vi "Lab Panel V5.22.vi"() -> ()   [LabVIEW 2013] (continued)
                      tunnel: w836 -> [_ w852]
                      tunnel: w835 -> [_ w851]
                      tunnel: w834 -> [_ w850]
                      tunnel: w833 -> [w843 w849]
                      tunnel: w832 -> [_ w847]
                      frame #0 {
                        n568 = Unbundle(w843) -> ("AMPS"=w846:dbl)  [unwired: 4 out]
                        n569 = call "Check For Amps on v1.vi"("ID"="LAB01-2", "amps"=w846) -> ("amps"=w844:bool)  [unwired: 9 in]
                      }
                      frame #1 {
                        n570 = case shown="True" w848 {
                          tunnel: w858 -> [_ w871]
                          tunnel: w857 -> [_ w870]
                          tunnel: w856 -> [_ w869]
                          tunnel: w855 -> [_ w868]
                          tunnel: w854 -> [_ w867]
                          tunnel: [errorcluster {"status"=FALSE, "code"=0, "source"=""} ("error out") w866] -> w853
                          tunnel: w852 -> [_ w865]
                          tunnel: w851 -> [_ w864]
                          tunnel: w850 -> [_ w863]
                          tunnel: w849 -> [_ w862]
                          tunnel: w847 -> [_ w861]
                          frame False {
                            w859 = FALSE
                            n571 = local write "RUN LAB01-2"(w859) -> ()
                            n572 = local write "run lab01-2"(w859) -> ()
                          }
                          frame True {
                            n573 = stacked-sequence {
                              seq-local: [w872 _ _ _ _] -> [_ w896 _ _ _]
                              tunnel: w871 -> [w877 _ _ _ _]
                              tunnel: w870 -> [w874 _ _ _ _]
                              tunnel: w869 -> [w887 _ _ _ _]
                              tunnel: w868 -> [w880 _ _ _ _]
                              tunnel: w867 -> [w875 _ _ _ _]
                              tunnel: [_ w891 _ _ _] -> w866
                              tunnel: w865 -> [_ _ _ w918 _]
                              tunnel: w864 -> [_ _ _ w917 _]
                              tunnel: w863 -> [_ _ _ w916 _]
                              tunnel: w862 -> [_ _ _ _ _]
                              tunnel: w861 -> [_ _ _ _ w931]
                              frame #0 {
                                w873 = "\\"
                                n574 = local read "SET LAB01-2"() -> (w882:T5)
                                n575 = case shown="\"CYCLE TEST\"" w887 {
                                tunnel: ["L01-2-CHART TEST-" "L01-2-CYCLE TEST-" "L01-2-T-RISE TEST-"] -> w883
                                frame "CHART TEST", Default {
                                }
                                frame "CYCLE TEST" {
                                }
                                frame "T-RISE TEST" {
                                }
                                }
                                n576 = Unbundle(w882) -> ("DESCRIPTION"=w881:string)  [unwired: 4 out]
                                n577 = Concatenate Strings(w877, "\\", w875, w873, w874, w873) -> (w884:string)
                                n578 = String To Path(string=w884) -> (path=w886:path)
                                n579 = Concatenate Strings(w884, w883, w881, "-", w880, ".tdms") -> (w872:string)
                                n580 = Create Folder(path (use dialog)=w886) -> (error out=w885:errorcluster)  [unwired: 2 in, 2 out]
                                n581 = call <vilib>:"Clear Errors.vi"("error in (no error)"=w885) -> ()  [unwired: 6 in, 1 out]
                                n582 = global write "Global 1.vi" "LAB01-2 FILE"(w872) -> ()
                              }
                              frame #1 {
                                (unwired) FALSE
                                n583 = String To Path(string=w896) -> (path=w892:path)
                                n584 = TDMS Open(6:FALSE, 10:T20."create or replace" ("operation (0:open)"), 11:w892) -> (0:w891:errorcluster, 3:→"TDMS LAB01-2":refnum<k34>)  [unwired: 4 in]
                              }
                              frame #2 {
                                n585 = local read "SET LAB01-2"() -> (w902:T5)
                                n586 = local read "TDMS LAB01-2"() -> (w913:refnum<k34>)
                                n587 = Build Array("Testers Name", "Description", "Set Test Cycles", "T-Rise minutes", "T-Rise Deg C") -> (w903:string[])
                                n588 = Unbundle(w902) -> ("NAME"=w901:string, "DESCRIPTION"=w900:string, "CYCLES"=w899:dbl, "T-RISE mins"=w898:dbl, "T-RISE deg C"=w897:dbl)
                                n589 = Number To Decimal String(number=w899) -> (decimal integer string=w912:string)  [unwired: 1 in]
                                n590 = Number To Decimal String(number=w898) -> (decimal integer string=w911:string)  [unwired: 1 in]
                                n591 = Number To Decimal String(number=w897) -> (decimal integer string=w910:string)  [unwired: 1 in]
                                n592 = Build Array(w901, w900, w912, w911, w910) -> (w909:string[])
                                n593 = TDMS Set Properties(5:w909, 7:w903, 11:w913) -> ()  [unwired: 3 in, 4 out]
                              }
                              frame #3 {
                                n594 = local read "DISP LAB01-2"() -> (w915:T4)
                                n595 = Concatenate Strings("LAB01-2  ", w918) -> (w919:string)
                                n596 = Two Button Dialog(message=w919, 1:w916, 2:w917) -> (T button?=w921:bool)
                                n597 = case shown="True" w921 {
                                tunnel: w915 -> [w928 w929]
                                tunnel: [w928 w929] -> w925
                                tunnel: [w927 w930] -> w924
                                tunnel: [w926 w930] -> w923
                                frame False {
                                n598 = Unbundle(w928) -> ("CYCLE"=w927:dbl, "MINS"=w926:dbl)  [unwired: 1 out]
                                }
                                frame True {
                                w930 = 0.0
                                }
                                }
                                n599 = Bundle(cluster=w925, "CYCLE"=w924, "MINS"=w923, "STATUS"="RUN") -> (w914:T4)
                                n600 = local write "DISP LAB01-2"(w914) -> ()
                              }
                              frame #4 {
                                n601 = local read "TEMP START LAB01-2"() -> (w933:cluster{"TL":dbl, "TN":dbl})
                                n602 = Bundle(cluster=w933, "TL"=w931, "TN"=w931) -> (w932:cluster{"TL":dbl, "TN":dbl})
                                n603 = local write "TEMP START LAB01-2"(w932) -> ()
                              }
                            }
                          }
                        }
                      }
                    }
                  }
                }
              }
              event "RUN LAB02-1": Value Change {
                n604 = event-data() -> ("NewVal"=w939:bool)  [unwired: 1 in, 5 out]
                n605 = local read "SIG LAB02-1"() -> (w935:T2)
                n606 = case shown="True" w939 {
                  tunnel: w945 -> [_ w983]
                  tunnel: w944 -> [_ w982]
                  tunnel: w942 -> [w947 w981]
                  tunnel: w943 -> [_ w980]
                  tunnel: w941 -> [_ w979]
                  tunnel: [w946 w978] -> w940
                  tunnel: w938 -> [_ w977]
                  tunnel: w937 -> [_ w976]
                  tunnel: w936 -> [_ w975]
                  tunnel: w935 -> [_ w974]
                  tunnel: w934 -> [_ w973]
                  frame False {
                    # "stop test"
                    n607 = stacked-sequence {
                      tunnel: w947 -> [w956 _]
                      tunnel: [w948 _] -> w946
                      frame #0 {
                        n608 = local read "DISP LAB02-1"() -> (w955:T4)
                        n609 = Unbundle(w955) -> ("CYCLE"=w953:dbl, "MINS"=w954:dbl)  [unwired: 1 out]
                        n610 = case shown="\"CYCLE TEST\"" w956 {
                          tunnel: w954 -> [_ _ w963]
                          tunnel: w953 -> [w961 w962 _]
                          tunnel: [w961 w962 w963] -> w952
                          frame "CHART TEST", Default {
                          }
                          frame "CYCLE TEST" {
                          }
                          frame "T-RISE TEST" {
                          }
                        }
                        n611 = local read "TDMS LAB02-1"() -> (w960:refnum<k34>)
                        n612 = Build Array("STOPPED") -> (w957:string[])
                        n613 = Build Array(w952) -> (w951:dbl[])
                        n614 = TDMS Write(0:w960, 5:"TEST RESULT", 7:w957, 9:w951) -> (4:w949:refnum<k34>, 15:w950:errorcluster)  [unwired: 2 in, 2 out]
                        n615 = TDMS Close(8:w950, 11:w949) -> (0:w948:errorcluster)  [unwired: 1 out]
                      }
                      frame #1 {
                        n616 = local read "DISP LAB02-1"() -> (w967:T4)
                        n617 = stacked-sequence {
                          tunnel: "LAB02-1" -> [w969 w971]
                          frame #0 {
                            n618 = call "sub vi - defrag tdms v1.vi"("panel id"=w969) -> ("error out"=w968:errorcluster)  [unwired: 10 in]
                            n619 = local write "data file error"(w968) -> ()
                          }
                          frame #1 {
                            n620 = local write "RESULT LAB02-1"(FALSE) -> ()
                            n621 = call "Save data file (stop) v3.vi"("panel id"=w971) -> ("network file save error"=w970:errorcluster)  [unwired: 9 in, 1 out]
                            n622 = local write "data file error"(w970) -> ()
                          }
                        }
                        n623 = Bundle(cluster=w967, "STATUS"="STOP") -> (w965:T4)  [unwired: 2 in]
                        n624 = local write "DISP LAB02-1"(w965) -> ()
                      }
                    }
                  }
                  frame True {
                    n625 = stacked-sequence {
                      seq-local: [w985 _] -> [_ w989]
                      tunnel: w983 -> [_ w999]
                      tunnel: w982 -> [_ w998]
                      tunnel: w981 -> [_ w997]
                      tunnel: w980 -> [_ w996]
                      tunnel: w979 -> [_ w995]
                      tunnel: [_ w994] -> w978
                      tunnel: w977 -> [_ w993]
                      tunnel: w976 -> [_ w992]
                      tunnel: w975 -> [_ w991]
                      tunnel: w974 -> [w984 w990]
                      tunnel: w973 -> [_ w988]
                      frame #0 {
                        n626 = Unbundle(w984) -> ("AMPS"=w987:dbl)  [unwired: 4 out]
                        n627 = call "Check For Amps on v1.vi"("ID"="LAB02-1", "amps"=w987) -> ("amps"=w985:bool)  [unwired: 9 in]
                      }
                      frame #1 {
                        n628 = case shown="True" w989 {
                          tunnel: w999 -> [_ w1012]
                          tunnel: w998 -> [_ w1011]
                          tunnel: w997 -> [_ w1010]
                          tunnel: w996 -> [_ w1009]
                          tunnel: w995 -> [_ w1008]
                          tunnel: [errorcluster {"status"=FALSE, "code"=0, "source"=""} ("error out") w1007] -> w994
                          tunnel: w993 -> [_ w1006]
                          tunnel: w992 -> [_ w1005]
                          tunnel: w991 -> [_ w1004]
                          tunnel: w990 -> [_ w1003]
                          tunnel: w988 -> [_ w1002]
                          frame False {
                            w1001 = FALSE
                            n629 = local write "RUN LAB02-1"(w1001) -> ()
                            n630 = local write "run lab02-1"(w1001) -> ()
                          }
                          frame True {
                            n631 = stacked-sequence {
                              seq-local: [w1013 _ _ _ _] -> [_ w1037 _ _ _]
                              tunnel: w1012 -> [w1018 _ _ _ _]
                              tunnel: w1011 -> [w1015 _ _ _ _]
                              tunnel: w1010 -> [w1028 _ _ _ _]
                              tunnel: w1009 -> [w1021 _ _ _ _]
                              tunnel: w1008 -> [w1016 _ _ _ _]
                              tunnel: [_ w1032 _ _ _] -> w1007
                              tunnel: w1006 -> [_ _ _ w1058 _]
                              tunnel: w1005 -> [_ _ _ w1057 _]
                              tunnel: w1004 -> [_ _ _ w1056 _]
                              tunnel: w1003 -> [_ _ _ _ _]
                              tunnel: w1002 -> [_ _ _ _ w1072]
                              frame #0 {
                                w1014 = "\\"
                                n632 = local read "SET LAB02-1"() -> (w1023:T5)
                                n633 = case shown="\"CYCLE TEST\"" w1028 {
                                tunnel: ["L02-1-CHART TEST-" "L02-1-CYCLE TEST-" "L02-1-T-RISE TEST-"] -> w1024
                                frame "CHART TEST", Default {
                                }
                                frame "CYCLE TEST" {
                                }
                                frame "T-RISE TEST" {
                                }
                                }
                                n634 = Unbundle(w1023) -> ("DESCRIPTION"=w1022:string)  [unwired: 4 out]
                                n635 = Concatenate Strings(w1018, "\\", w1016, w1014, w1015, w1014) -> (w1025:string)
                                n636 = String To Path(string=w1025) -> (path=w1027:path)
                                n637 = Concatenate Strings(w1025, w1024, w1022, "-", w1021, ".tdms") -> (w1013:string)
                                n638 = Create Folder(path (use dialog)=w1027) -> (error out=w1026:errorcluster)  [unwired: 2 in, 2 out]
                                n639 = global write "Global 1.vi" "LAB02-1 FILE"(w1013) -> ()
                                n640 = call <vilib>:"Clear Errors.vi"("error in (no error)"=w1026) -> ()  [unwired: 6 in, 1 out]
                              }
                              frame #1 {
                                (unwired) FALSE
                                n641 = String To Path(string=w1037) -> (path=w1033:path)
                                n642 = TDMS Open(6:FALSE, 10:T20."create or replace" ("operation (0:open)"), 11:w1033) -> (0:w1032:errorcluster, 3:→"TDMS LAB02-1":refnum<k34>)  [unwired: 4 in]
                              }
                              frame #2 {
                                n643 = local read "SET LAB02-1"() -> (w1043:T5)
                                n644 = local read "TDMS LAB02-1"() -> (w1054:refnum<k34>)
                                n645 = Build Array("Testers Name", "Description", "Set Test Cycles", "T-Rise minutes", "T-Rise Deg C") -> (w1044:string[])
                                n646 = Unbundle(w1043) -> ("NAME"=w1042:string, "DESCRIPTION"=w1041:string, "CYCLES"=w1040:dbl, "T-RISE mins"=w1039:dbl, "T-RISE deg C"=w1038:dbl)
                                n647 = Number To Decimal String(number=w1040) -> (decimal integer string=w1053:string)  [unwired: 1 in]
                                n648 = Number To Decimal String(number=w1039) -> (decimal integer string=w1052:string)  [unwired: 1 in]
                                n649 = Number To Decimal String(number=w1038) -> (decimal integer string=w1051:string)  [unwired: 1 in]
                                n650 = Build Array(w1042, w1041, w1053, w1052, w1051) -> (w1050:string[])
                                n651 = TDMS Set Properties(5:w1050, 7:w1044, 11:w1054) -> ()  [unwired: 3 in, 4 out]
                              }
                              frame #3 {
                                n652 = local read "DISP LAB02-1"() -> (w1059:T4)
                                n653 = Concatenate Strings("LAB02-1  ", w1058) -> (w1060:string)
                                n654 = Two Button Dialog(message=w1060, 1:w1056, 2:w1057) -> (T button?=w1062:bool)
                                n655 = case shown="True" w1062 {
                                tunnel: w1059 -> [w1069 w1070]
                                tunnel: [w1069 w1070] -> w1066
                                tunnel: [w1068 w1071] -> w1065
                                tunnel: [w1067 w1071] -> w1064
                                frame False {
                                n656 = Unbundle(w1069) -> ("CYCLE"=w1068:dbl, "MINS"=w1067:dbl)  [unwired: 1 out]
                                }
                                frame True {
                                w1071 = 0.0
                                }
                                }
                                n657 = Bundle(cluster=w1066, "CYCLE"=w1065, "MINS"=w1064, "STATUS"="RUN") -> (w1055:T4)
                                n658 = local write "DISP LAB02-1"(w1055) -> ()
                              }
                              frame #4 {
                                n659 = local read "TEMP START LAB02-1"() -> (w1074:cluster{"TL":dbl, "TN":dbl})
                                n660 = Bundle(cluster=w1074, "TL"=w1072, "TN"=w1072) -> (w1073:cluster{"TL":dbl, "TN":dbl})
                                n661 = local write "TEMP START LAB02-1"(w1073) -> ()
                              }
                            }
                          }
                        }
                      }
                    }
                  }
                }
                n662 = local write "run lab02-1"(w939) -> ()
              }
              event "RUN LAB02-2": Value Change {
                n663 = event-data() -> ("NewVal"=w1079:bool)  [unwired: 1 in, 5 out]
                n664 = local write "run lab02-2"(w1079) -> ()
                n665 = case shown="True" w1079 {
                  tunnel: w1085 -> [_ w1123]
                  tunnel: w1084 -> [_ w1122]
                  tunnel: w1082 -> [w1087 w1121]
                  tunnel: w1083 -> [_ w1120]
                  tunnel: w1081 -> [_ w1119]
                  tunnel: [w1086 w1118] -> w1080
                  tunnel: w1078 -> [_ w1117]
                  tunnel: w1077 -> [_ w1116]
                  tunnel: w1076 -> [_ w1115]
                  tunnel: w1075 -> [_ w1113]
                  frame False {
                    # "stop test"
                    n666 = stacked-sequence {
                      tunnel: w1087 -> [w1096 _]
                      tunnel: [w1088 _] -> w1086
                      frame #0 {
                        n667 = local read "DISP LAB02-2"() -> (w1095:T4)
                        n668 = Unbundle(w1095) -> ("CYCLE"=w1093:dbl, "MINS"=w1094:dbl)  [unwired: 1 out]
                        n669 = case shown="\"CYCLE TEST\"" w1096 {
                          tunnel: w1094 -> [_ _ w1103]
                          tunnel: w1093 -> [w1101 w1102 _]
                          tunnel: [w1101 w1102 w1103] -> w1092
                          frame "CHART TEST", Default {
                          }
                          frame "CYCLE TEST" {
                          }
                          frame "T-RISE TEST" {
                          }
                        }
                        n670 = local read "TDMS LAB02-2"() -> (w1100:refnum<k34>)
                        n671 = Build Array("STOPPED") -> (w1097:string[])
                        n672 = Build Array(w1092) -> (w1091:dbl[])
                        n673 = TDMS Write(0:w1100, 5:"TEST RESULT", 7:w1097, 9:w1091) -> (4:w1089:refnum<k34>, 15:w1090:errorcluster)  [unwired: 2 in, 2 out]
                        n674 = TDMS Close(8:w1090, 11:w1089) -> (0:w1088:errorcluster)  [unwired: 1 out]
                      }
                      frame #1 {
                        n675 = local read "DISP LAB02-2"() -> (w1107:T4)
                        n676 = stacked-sequence {
                          tunnel: "LAB02-2" -> [w1109 w1111]
                          frame #0 {
                            n677 = call "sub vi - defrag tdms v1.vi"("panel id"=w1109) -> ("error out"=w1108:errorcluster)  [unwired: 10 in]
                            n678 = local write "data file error"(w1108) -> ()
                          }
                          frame #1 {
                            n679 = call "Save data file (stop) v3.vi"("panel id"=w1111) -> ("network file save error"=w1110:errorcluster)  [unwired: 9 in, 1 out]
                            n680 = local write "RESULT LAB02-2"(FALSE) -> ()
                            n681 = local write "data file error"(w1110) -> ()
                          }
                        }
                        n682 = Bundle(cluster=w1107, "STATUS"="STOP") -> (w1105:T4)  [unwired: 2 in]
                        n683 = local write "DISP LAB02-2"(w1105) -> ()
                      }
                    }
                  }
                  frame True {
                    n684 = local read "SIG LAB02-2"() -> (w1114:T2)
                    n685 = stacked-sequence {
                      seq-local: [w1125 _] -> [_ w1129]
                      tunnel: w1123 -> [_ w1139]
                      tunnel: w1122 -> [_ w1138]
                      tunnel: w1121 -> [_ w1137]
                      tunnel: w1120 -> [_ w1136]
                      tunnel: w1119 -> [_ w1135]
                      tunnel: [_ w1134] -> w1118
                      tunnel: w1117 -> [_ w1133]
                      tunnel: w1116 -> [_ w1132]
                      tunnel: w1115 -> [_ w1131]
                      tunnel: w1114 -> [w1124 w1130]
                      tunnel: w1113 -> [_ w1128]
                      frame #0 {
                        n686 = Unbundle(w1124) -> ("AMPS"=w1127:dbl)  [unwired: 4 out]
                        n687 = call "Check For Amps on v1.vi"("ID"="LAB02-2", "amps"=w1127) -> ("amps"=w1125:bool)  [unwired: 9 in]
                      }
                      frame #1 {
                        n688 = case shown="True" w1129 {
                          tunnel: w1139 -> [_ w1152]
                          tunnel: w1138 -> [_ w1151]
                          tunnel: w1137 -> [_ w1150]
                          tunnel: w1136 -> [_ w1149]
                          tunnel: w1135 -> [_ w1148]
                          tunnel: [errorcluster {"status"=FALSE, "code"=0, "source"=""} ("error out") w1147] -> w1134
                          tunnel: w1133 -> [_ w1146]
                          tunnel: w1132 -> [_ w1145]
                          tunnel: w1131 -> [_ w1144]
                          tunnel: w1130 -> [_ w1143]
                          tunnel: w1128 -> [_ w1142]
                          frame False {
                            w1140 = FALSE
                            n689 = local write "RUN LAB02-2"(w1140) -> ()
                            n690 = local write "run lab02-2"(w1140) -> ()
                          }
                          frame True {
                            n691 = stacked-sequence {
                              seq-local: [w1153 _ _ _ _] -> [_ w1177 _ _ _]
                              tunnel: w1152 -> [w1158 _ _ _ _]
                              tunnel: w1151 -> [w1155 _ _ _ _]
                              tunnel: w1150 -> [w1168 _ _ _ _]
                              tunnel: w1149 -> [w1161 _ _ _ _]
                              tunnel: w1148 -> [w1156 _ _ _ _]
                              tunnel: [_ w1172 _ _ _] -> w1147
                              tunnel: w1146 -> [_ _ _ w1198 _]
                              tunnel: w1145 -> [_ _ _ w1197 _]
                              tunnel: w1144 -> [_ _ _ w1196 _]
                              tunnel: w1143 -> [_ _ _ _ _]
                              tunnel: w1142 -> [_ _ _ _ w1212]
                              frame #0 {
                                w1154 = "\\"
                                n692 = local read "SET LAB02-2"() -> (w1163:T5)
                                n693 = case shown="\"CYCLE TEST\"" w1168 {
                                tunnel: ["L02-2-CHART TEST-" "L02-2-CYCLE TEST-" "L02-2-T-RISE TEST-"] -> w1164
                                frame "CHART TEST", Default {
                                }
                                frame "CYCLE TEST" {
                                }
                                frame "T-RISE TEST" {
                                }
                                }
                                n694 = Unbundle(w1163) -> ("DESCRIPTION"=w1162:string)  [unwired: 4 out]
                                n695 = Concatenate Strings(w1158, "\\", w1156, w1154, w1155, w1154) -> (w1165:string)
                                n696 = String To Path(string=w1165) -> (path=w1167:path)
                                n697 = Concatenate Strings(w1165, w1164, w1162, "-", w1161, ".tdms") -> (w1153:string)
                                n698 = Create Folder(path (use dialog)=w1167) -> (error out=w1166:errorcluster)  [unwired: 2 in, 2 out]
                                n699 = global write "Global 1.vi" "LAB02-2 FILE"(w1153) -> ()
                                n700 = call <vilib>:"Clear Errors.vi"("error in (no error)"=w1166) -> ()  [unwired: 6 in, 1 out]
                              }
                              frame #1 {
                                (unwired) FALSE
                                n701 = String To Path(string=w1177) -> (path=w1173:path)
                                n702 = TDMS Open(6:FALSE, 10:T20."create or replace" ("operation (0:open)"), 11:w1173) -> (0:w1172:errorcluster, 3:→"TDMS LAB02-2":refnum<k34>)  [unwired: 4 in]
                              }
                              frame #2 {
                                n703 = local read "SET LAB02-2"() -> (w1183:T5)
                                n704 = local read "TDMS LAB02-2"() -> (w1194:refnum<k34>)
                                n705 = Build Array("Testers Name", "Description", "Set Test Cycles", "T-Rise minutes", "T-Rise Deg C") -> (w1184:string[])
                                n706 = Unbundle(w1183) -> ("NAME"=w1182:string, "DESCRIPTION"=w1181:string, "CYCLES"=w1180:dbl, "T-RISE mins"=w1179:dbl, "T-RISE deg C"=w1178:dbl)
                                n707 = Number To Decimal String(number=w1180) -> (decimal integer string=w1193:string)  [unwired: 1 in]
                                n708 = Number To Decimal String(number=w1179) -> (decimal integer string=w1192:string)  [unwired: 1 in]
                                n709 = Number To Decimal String(number=w1178) -> (decimal integer string=w1191:string)  [unwired: 1 in]
                                n710 = Build Array(w1182, w1181, w1193, w1192, w1191) -> (w1190:string[])
                                n711 = TDMS Set Properties(5:w1190, 7:w1184, 11:w1194) -> ()  [unwired: 3 in, 4 out]
                              }
                              frame #3 {
                                n712 = local read "DISP LAB02-2"() -> (w1199:T4)
                                n713 = Concatenate Strings("LAB02-2  ", w1198) -> (w1200:string)
                                n714 = Two Button Dialog(message=w1200, 1:w1196, 2:w1197) -> (T button?=w1202:bool)
                                n715 = case shown="True" w1202 {
                                tunnel: w1199 -> [w1209 w1210]
                                tunnel: [w1209 w1210] -> w1206
                                tunnel: [w1208 w1211] -> w1205
                                tunnel: [w1207 w1211] -> w1204
                                frame False {
                                n716 = Unbundle(w1209) -> ("CYCLE"=w1208:dbl, "MINS"=w1207:dbl)  [unwired: 1 out]
                                }
                                frame True {
                                w1211 = 0.0
                                }
                                }
                                n717 = Bundle(cluster=w1206, "CYCLE"=w1205, "MINS"=w1204, "STATUS"="RUN") -> (w1195:T4)
                                n718 = local write "DISP LAB02-2"(w1195) -> ()
                              }
                              frame #4 {
                                n719 = local read "TEMP START LAB02-2"() -> (w1214:cluster{"TL":dbl, "TN":dbl})
                                n720 = Bundle(cluster=w1214, "TL"=w1212, "TN"=w1212) -> (w1213:cluster{"TL":dbl, "TN":dbl})
                                n721 = local write "TEMP START LAB02-2"(w1213) -> ()
                              }
                            }
                          }
                        }
                      }
                    }
                  }
                }
              }
              event "RUN LAB03-1": Value Change {
                n722 = event-data() -> ("NewVal"=w1219:bool)  [unwired: 1 in, 5 out]
                n723 = local write "run lab03-1"(w1219) -> ()
                n724 = case shown="True" w1219 {
                  tunnel: w1225 -> [_ w1263]
                  tunnel: w1224 -> [_ w1262]
                  tunnel: w1222 -> [w1227 w1261]
                  tunnel: w1223 -> [_ w1260]
                  tunnel: w1221 -> [_ w1259]
                  tunnel: [w1226 w1258] -> w1220
                  tunnel: w1218 -> [_ w1257]
                  tunnel: w1217 -> [_ w1256]
                  tunnel: w1216 -> [_ w1255]
                  tunnel: w1215 -> [_ w1253]
                  frame False {
                    # "stop test"
                    n725 = stacked-sequence {
                      tunnel: w1227 -> [w1236 _]
                      tunnel: [w1228 _] -> w1226
                      frame #0 {
                        n726 = local read "DISP LAB03-1"() -> (w1235:T4)
                        n727 = Unbundle(w1235) -> ("CYCLE"=w1233:dbl, "MINS"=w1234:dbl)  [unwired: 1 out]
                        n728 = case shown="\"CYCLE TEST\"" w1236 {
                          tunnel: w1234 -> [_ _ w1243]
                          tunnel: w1233 -> [w1241 w1242 _]
                          tunnel: [w1241 w1242 w1243] -> w1232
                          frame "CHART TEST", Default {
                          }
                          frame "CYCLE TEST" {
                          }
                          frame "T-RISE TEST" {
                          }
                        }
                        n729 = local read "TDMS LAB03-1"() -> (w1240:refnum<k34>)
                        n730 = Build Array("STOPPED") -> (w1237:string[])
                        n731 = Build Array(w1232) -> (w1231:dbl[])
                        n732 = TDMS Write(0:w1240, 5:"TEST RESULT", 7:w1237, 9:w1231) -> (4:w1229:refnum<k34>, 15:w1230:errorcluster)  [unwired: 2 in, 2 out]
                        n733 = TDMS Close(8:w1230, 11:w1229) -> (0:w1228:errorcluster)  [unwired: 1 out]
                      }
                      frame #1 {
                        n734 = local read "DISP LAB03-1"() -> (w1247:T4)
                        n735 = stacked-sequence {
                          tunnel: "LAB03-1" -> [w1249 w1251]
                          frame #0 {
                            n736 = call "sub vi - defrag tdms v1.vi"("panel id"=w1249) -> ("error out"=w1248:errorcluster)  [unwired: 10 in]
                            n737 = local write "data file error"(w1248) -> ()
                          }
                          frame #1 {
                            n738 = call "Save data file (stop) v3.vi"("panel id"=w1251) -> ("network file save error"=w1250:errorcluster)  [unwired: 9 in, 1 out]
                            n739 = local write "RESULT LAB03-1"(FALSE) -> ()
                            n740 = local write "data file error"(w1250) -> ()
                          }
                        }
                        n741 = Bundle(cluster=w1247, "STATUS"="STOP") -> (w1245:T4)  [unwired: 2 in]
                        n742 = local write "DISP LAB03-1"(w1245) -> ()
                      }
                    }
                  }
                  frame True {
                    n743 = local read "SIG LAB03-1"() -> (w1254:T2)
                    n744 = stacked-sequence {
                      seq-local: [w1265 _] -> [_ w1269]
                      tunnel: w1263 -> [_ w1279]
                      tunnel: w1262 -> [_ w1278]
                      tunnel: w1261 -> [_ w1277]
                      tunnel: w1260 -> [_ w1276]
                      tunnel: w1259 -> [_ w1275]
                      tunnel: [_ w1274] -> w1258
                      tunnel: w1257 -> [_ w1273]
                      tunnel: w1256 -> [_ w1272]
                      tunnel: w1255 -> [_ w1271]
                      tunnel: w1254 -> [w1264 w1270]
                      tunnel: w1253 -> [_ w1268]
                      frame #0 {
                        n745 = Unbundle(w1264) -> ("AMPS"=w1267:dbl)  [unwired: 4 out]
                        n746 = call "Check For Amps on v1.vi"("ID"="LAB03-1", "amps"=w1267) -> ("amps"=w1265:bool)  [unwired: 9 in]
                      }
                      frame #1 {
                        n747 = case shown="True" w1269 {
                          tunnel: w1279 -> [_ w1292]
                          tunnel: w1278 -> [_ w1291]
                          tunnel: w1277 -> [_ w1290]
                          tunnel: w1276 -> [_ w1289]
                          tunnel: w1275 -> [_ w1288]
                          tunnel: [errorcluster {"status"=FALSE, "code"=0, "source"=""} ("error out") w1287] -> w1274
                          tunnel: w1273 -> [_ w1286]
                          tunnel: w1272 -> [_ w1285]
                          tunnel: w1271 -> [_ w1284]
                          tunnel: w1270 -> [_ w1283]
                          tunnel: w1268 -> [_ w1282]
                          frame False {
                            w1280 = FALSE
                            n748 = local write "RUN LAB03-1"(w1280) -> ()
                            n749 = local write "run lab03-1"(w1280) -> ()
                          }
                          frame True {
                            n750 = stacked-sequence {
                              seq-local: [w1293 _ _ _ _] -> [_ w1317 _ _ _]
                              tunnel: w1292 -> [w1298 _ _ _ _]
                              tunnel: w1291 -> [w1295 _ _ _ _]
                              tunnel: w1290 -> [w1308 _ _ _ _]
                              tunnel: w1289 -> [w1301 _ _ _ _]
                              tunnel: w1288 -> [w1296 _ _ _ _]
                              tunnel: [_ w1312 _ _ _] -> w1287
                              tunnel: w1286 -> [_ _ _ w1337 _]
                              tunnel: w1285 -> [_ _ _ w1336 _]
                              tunnel: w1284 -> [_ _ _ w1335 _]
                              tunnel: w1283 -> [_ _ _ _ _]
                              tunnel: w1282 -> [_ _ _ _ w1352]
                              frame #0 {
                                w1294 = "\\"
                                n751 = local read "SET LAB03-1"() -> (w1303:T5)
                                n752 = case shown="\"T-RISE TEST\"" w1308 {
                                tunnel: ["L03-1-CHART TEST-" "L03-1-CYCLE TEST-" "L03-1-T-RISE TEST-"] -> w1304
                                frame "CHART TEST", Default {
                                }
                                frame "CYCLE TEST" {
                                }
                                frame "T-RISE TEST" {
                                }
                                }
                                n753 = Unbundle(w1303) -> ("DESCRIPTION"=w1302:string)  [unwired: 4 out]
                                n754 = Concatenate Strings(w1298, "\\", w1296, w1294, w1295, w1294) -> (w1305:string)
                                n755 = String To Path(string=w1305) -> (path=w1307:path)
                                n756 = Concatenate Strings(w1305, w1304, w1302, "-", w1301, ".tdms") -> (w1293:string)
                                n757 = Create Folder(path (use dialog)=w1307) -> (error out=w1306:errorcluster)  [unwired: 2 in, 2 out]
                                n758 = global write "Global 1.vi" "LAB03-1 FILE"(w1293) -> ()
                                n759 = call <vilib>:"Clear Errors.vi"("error in (no error)"=w1306) -> ()  [unwired: 6 in, 1 out]
                              }
                              frame #1 {
                                (unwired) FALSE
                                n760 = String To Path(string=w1317) -> (path=w1313:path)
                                n761 = TDMS Open(6:FALSE, 10:T20."create or replace" ("operation (0:open)"), 11:w1313) -> (0:w1312:errorcluster, 3:→"TDMS LAB03-1":refnum<k34>)  [unwired: 4 in]
                              }
                              frame #2 {
                                n762 = local read "SET LAB03-1"() -> (w1323:T5)
                                n763 = local read "TDMS LAB03-1"() -> (w1334:refnum<k34>)
                                n764 = Build Array("Testers Name", "Description", "Set Test Cycles", "T-Rise minutes", "T-Rise Deg C") -> (w1324:string[])
                                n765 = Unbundle(w1323) -> ("NAME"=w1322:string, "DESCRIPTION"=w1321:string, "CYCLES"=w1320:dbl, "T-RISE mins"=w1319:dbl, "T-RISE deg C"=w1318:dbl)
                                n766 = Number To Decimal String(number=w1320) -> (decimal integer string=w1333:string)  [unwired: 1 in]
                                n767 = Number To Decimal String(number=w1319) -> (decimal integer string=w1332:string)  [unwired: 1 in]
                                n768 = Number To Decimal String(number=w1318) -> (decimal integer string=w1331:string)  [unwired: 1 in]
                                n769 = Build Array(w1322, w1321, w1333, w1332, w1331) -> (w1330:string[])
                                n770 = TDMS Set Properties(5:w1330, 7:w1324, 11:w1334) -> ()  [unwired: 3 in, 4 out]
                              }
                              frame #3 {
                                n771 = local read "DISP LAB03-1"() -> (w1339:T4)
                                n772 = Concatenate Strings("LAB03-1  ", w1337) -> (w1340:string)
                                n773 = Two Button Dialog(message=w1340, 1:w1335, 2:w1336) -> (T button?=w1342:bool)
                                n774 = case shown="True" w1342 {
                                tunnel: w1339 -> [w1349 w1350]
                                tunnel: [w1349 w1350] -> w1346
                                tunnel: [w1348 w1351] -> w1345
                                tunnel: [w1347 w1351] -> w1344
                                frame False {
                                n775 = Unbundle(w1349) -> ("CYCLE"=w1348:dbl, "MINS"=w1347:dbl)  [unwired: 1 out]
                                }
                                frame True {
                                w1351 = 0.0
                                }
                                }
                                n776 = Bundle(cluster=w1346, "CYCLE"=w1345, "MINS"=w1344, "STATUS"="RUN") -> (w1338:T4)
                                n777 = local write "DISP LAB03-1"(w1338) -> ()
                              }
                              frame #4 {
                                n778 = local read "TEMP START LAB03-1"() -> (w1354:cluster{"TL":dbl, "TN":dbl})
                                n779 = Bundle(cluster=w1354, "TL"=w1352, "TN"=w1352) -> (w1353:cluster{"TL":dbl, "TN":dbl})
                                n780 = local write "TEMP START LAB03-1"(w1353) -> ()
                              }
                            }
                          }
                        }
                      }
                    }
                  }
                }
              }
              event "RUN LAB03-2": Value Change {
                n781 = event-data() -> ("NewVal"=w1359:bool)  [unwired: 1 in, 5 out]
                n782 = local write "run lab03-2"(w1359) -> ()
                n783 = case shown="True" w1359 {
                  tunnel: w1365 -> [_ w1403]
                  tunnel: w1364 -> [_ w1402]
                  tunnel: w1362 -> [w1367 w1401]
                  tunnel: w1363 -> [_ w1400]
                  tunnel: w1361 -> [_ w1399]
                  tunnel: [w1366 w1398] -> w1360
                  tunnel: w1358 -> [_ w1397]
                  tunnel: w1357 -> [_ w1396]
                  tunnel: w1356 -> [_ w1395]
                  tunnel: w1355 -> [_ w1393]
                  frame False {
                    # "stop test"
                    n784 = stacked-sequence {
                      tunnel: w1367 -> [w1376 _]
                      tunnel: [w1368 _] -> w1366
                      frame #0 {
                        n785 = local read "DISP LAB03-2"() -> (w1375:T4)
                        n786 = Unbundle(w1375) -> ("CYCLE"=w1373:dbl, "MINS"=w1374:dbl)  [unwired: 1 out]
                        n787 = case shown="\"CYCLE TEST\"" w1376 {
                          tunnel: w1374 -> [_ _ w1383]
                          tunnel: w1373 -> [w1381 w1382 _]
                          tunnel: [w1381 w1382 w1383] -> w1372
                          frame "CHART TEST", Default {
                          }
                          frame "CYCLE TEST" {
                          }
                          frame "T-RISE TEST" {
                          }
                        }
                        n788 = local read "TDMS LAB03-2"() -> (w1380:refnum<k34>)
                        n789 = Build Array("STOPPED") -> (w1377:string[])
                        n790 = Build Array(w1372) -> (w1371:dbl[])
                        n791 = TDMS Write(0:w1380, 5:"TEST RESULT", 7:w1377, 9:w1371) -> (4:w1369:refnum<k34>, 15:w1370:errorcluster)  [unwired: 2 in, 2 out]
                        n792 = TDMS Close(8:w1370, 11:w1369) -> (0:w1368:errorcluster)  [unwired: 1 out]
                      }
                      frame #1 {
                        n793 = local read "DISP LAB03-2"() -> (w1387:T4)
                        n794 = stacked-sequence {
                          tunnel: "LAB03-2" -> [w1389 w1391]
                          frame #0 {
                            n795 = call "sub vi - defrag tdms v1.vi"("panel id"=w1389) -> ("error out"=w1388:errorcluster)  [unwired: 10 in]
                            n796 = local write "data file error"(w1388) -> ()
                          }
                          frame #1 {
                            n797 = call "Save data file (stop) v3.vi"("panel id"=w1391) -> ("network file save error"=w1390:errorcluster)  [unwired: 9 in, 1 out]
                            n798 = local write "RESULT LAB03-2"(FALSE) -> ()
                            n799 = local write "data file error"(w1390) -> ()
                          }
                        }
                        n800 = Bundle(cluster=w1387, "STATUS"="STOP") -> (w1385:T4)  [unwired: 2 in]
                        n801 = local write "DISP LAB03-2"(w1385) -> ()
                      }
                    }
                  }
                  frame True {
                    n802 = local read "SIG LAB03-2"() -> (w1394:T2)
                    n803 = stacked-sequence {
                      seq-local: [w1405 _] -> [_ w1409]
                      tunnel: w1403 -> [_ w1419]
                      tunnel: w1402 -> [_ w1418]
                      tunnel: w1401 -> [_ w1417]
                      tunnel: w1400 -> [_ w1416]
                      tunnel: w1399 -> [_ w1415]
                      tunnel: [_ w1414] -> w1398
                      tunnel: w1397 -> [_ w1413]
                      tunnel: w1396 -> [_ w1412]
                      tunnel: w1395 -> [_ w1411]
                      tunnel: w1394 -> [w1404 w1410]
                      tunnel: w1393 -> [_ w1408]
                      frame #0 {
                        n804 = Unbundle(w1404) -> ("AMPS"=w1407:dbl)  [unwired: 4 out]
                        n805 = call "Check For Amps on v1.vi"("ID"="LAB03-2", "amps"=w1407) -> ("amps"=w1405:bool)  [unwired: 9 in]
                      }
                      frame #1 {
                        n806 = case shown="True" w1409 {
                          tunnel: w1419 -> [_ w1432]
                          tunnel: w1418 -> [_ w1431]
                          tunnel: w1417 -> [_ w1430]
                          tunnel: w1416 -> [_ w1429]
                          tunnel: w1415 -> [_ w1428]
                          tunnel: [errorcluster {"status"=FALSE, "code"=0, "source"=""} ("error out") w1427] -> w1414
                          tunnel: w1413 -> [_ w1426]
                          tunnel: w1412 -> [_ w1425]
                          tunnel: w1411 -> [_ w1424]
                          tunnel: w1410 -> [_ w1423]
                          tunnel: w1408 -> [_ w1422]
                          frame False {
                            w1420 = FALSE
                            n807 = local write "RUN LAB03-2"(w1420) -> ()
                            n808 = local write "run lab03-2"(w1420) -> ()
                          }
                          frame True {
                            n809 = stacked-sequence {
                              seq-local: [w1433 _ _ _ _] -> [_ w1457 _ _ _]
                              tunnel: w1432 -> [w1438 _ _ _ _]
                              tunnel: w1431 -> [w1435 _ _ _ _]
                              tunnel: w1430 -> [w1448 _ _ _ _]
                              tunnel: w1429 -> [w1441 _ _ _ _]
                              tunnel: w1428 -> [w1436 _ _ _ _]
                              tunnel: [_ w1452 _ _ _] -> w1427
                              tunnel: w1426 -> [_ _ _ w1478 _]
                              tunnel: w1425 -> [_ _ _ w1477 _]
                              tunnel: w1424 -> [_ _ _ w1476 _]
                              tunnel: w1423 -> [_ _ _ _ _]
                              tunnel: w1422 -> [_ _ _ _ w1492]
                              frame #0 {
                                w1434 = "\\"
                                n810 = local read "SET LAB03-2"() -> (w1443:T5)
                                n811 = case shown="\"T-RISE TEST\"" w1448 {
                                tunnel: ["L03-2-CHART TEST-" "L03-2-CYCLE TEST-" "L03-2-T-RISE TEST-"] -> w1444
                                frame "CHART TEST", Default {
                                }
                                frame "CYCLE TEST" {
                                }
                                frame "T-RISE TEST" {
                                }
                                }
                                n812 = Unbundle(w1443) -> ("DESCRIPTION"=w1442:string)  [unwired: 4 out]
                                n813 = Concatenate Strings(w1438, "\\", w1436, w1434, w1435, w1434) -> (w1445:string)
                                n814 = String To Path(string=w1445) -> (path=w1447:path)
                                n815 = Concatenate Strings(w1445, w1444, w1442, "-", w1441, ".tdms") -> (w1433:string)
                                n816 = Create Folder(path (use dialog)=w1447) -> (error out=w1446:errorcluster)  [unwired: 2 in, 2 out]
                                n817 = global write "Global 1.vi" "LAB03-2 FILE"(w1433) -> ()
                                n818 = call <vilib>:"Clear Errors.vi"("error in (no error)"=w1446) -> ()  [unwired: 6 in, 1 out]
                              }
                              frame #1 {
                                (unwired) FALSE
                                n819 = String To Path(string=w1457) -> (path=w1453:path)
                                n820 = TDMS Open(6:FALSE, 10:T20."create or replace" ("operation (0:open)"), 11:w1453) -> (0:w1452:errorcluster, 3:→"TDMS LAB03-2":refnum<k34>)  [unwired: 4 in]
                              }
                              frame #2 {
                                n821 = local read "SET LAB03-2"() -> (w1463:T5)
                                n822 = local read "TDMS LAB03-2"() -> (w1474:refnum<k34>)
                                n823 = Build Array("Testers Name", "Description", "Set Test Cycles", "T-Rise minutes", "T-Rise Deg C") -> (w1464:string[])
                                n824 = Unbundle(w1463) -> ("NAME"=w1462:string, "DESCRIPTION"=w1461:string, "CYCLES"=w1460:dbl, "T-RISE mins"=w1459:dbl, "T-RISE deg C"=w1458:dbl)
                                n825 = Number To Decimal String(number=w1460) -> (decimal integer string=w1473:string)  [unwired: 1 in]
                                n826 = Number To Decimal String(number=w1459) -> (decimal integer string=w1472:string)  [unwired: 1 in]
                                n827 = Number To Decimal String(number=w1458) -> (decimal integer string=w1471:string)  [unwired: 1 in]
                                n828 = Build Array(w1462, w1461, w1473, w1472, w1471) -> (w1470:string[])
                                n829 = TDMS Set Properties(5:w1470, 7:w1464, 11:w1474) -> ()  [unwired: 3 in, 4 out]
                              }
                              frame #3 {
                                n830 = local read "DISP LAB03-2"() -> (w1479:T4)
                                n831 = Concatenate Strings("LAB03-2  ", w1478) -> (w1480:string)
                                n832 = Two Button Dialog(message=w1480, 1:w1476, 2:w1477) -> (T button?=w1482:bool)
                                n833 = case shown="True" w1482 {
                                tunnel: w1479 -> [w1489 w1490]
                                tunnel: [w1489 w1490] -> w1486
                                tunnel: [w1488 w1491] -> w1485
                                tunnel: [w1487 w1491] -> w1484
                                frame False {
                                n834 = Unbundle(w1489) -> ("CYCLE"=w1488:dbl, "MINS"=w1487:dbl)  [unwired: 1 out]
                                }
                                frame True {
                                w1491 = 0.0
                                }
                                }
                                n835 = Bundle(cluster=w1486, "CYCLE"=w1485, "MINS"=w1484, "STATUS"="RUN") -> (w1475:T4)
